vi "Set Value.vi"(8 "error in":errorcluster, 10 "Image":variant[][](array[variant]), 11 "Base Graph in":refnum<class "Base Graph.lvclass">) -> (0 "error out":errorcluster, 3 "Base Graph out":refnum<class "Base Graph.lvclass">)   [LabVIEW 2023, in "Base Graph.lvclass"]
uses:
  Base Graph.lvclass
  Base Graph.lvclass/Base Graph.ctl
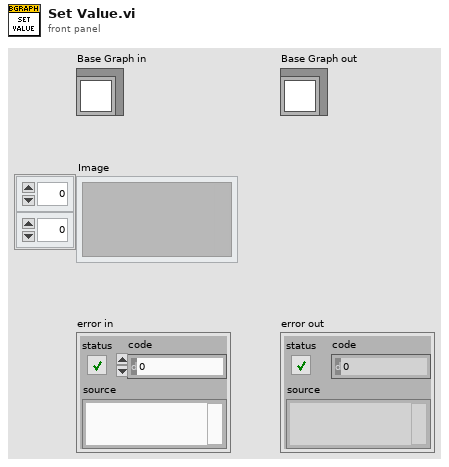
[diagram p1: front panel]
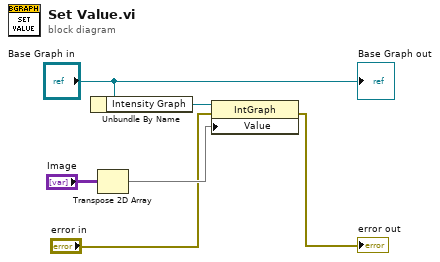
[diagram p0: block diagram]
diagram:
  n1 = Unbundle By Name("Base Graph in") -> ("Intensity Graph"=w5:refnum<vi>)
  n2 = Transpose 2D Array(2D array="Image") -> (transposed array=w4:variant[][])
  n3 = property class="IntGraph"(reference=w5, error in="error in", "Value"=w4) -> (error out=→"error out":errorcluster)  [unwired: 1 out]
  "Base Graph out" <- "Base Graph in"
